vi "Verify Cancel.vi"(11 "Calling VI":refnum<vi>) -> (0 "error out":errorcluster, 2 "Close IE":bool)   [LabVIEW 2020, in "lv_icon.lvlib"]
doc: "Checks if there were changes to the icon and allows the user to select to keep or discord those changes or to return to the Icon Editor."
uses:
  lv_icon.lvlib
  History/History.lvclass
  Controls/Undo Redo Action.ctl
panel:
  in  "Cancel":bool
  in  "Discard":bool
  in  "Apply":bool
  # "The icon has unapplied changes.\nDo you want to apply or discard the changes?"
  # "Apply the changes to the VI"
  # "Changes are discarded and the Icon Editor will be closed"
  # "Return to the Icon Editor"
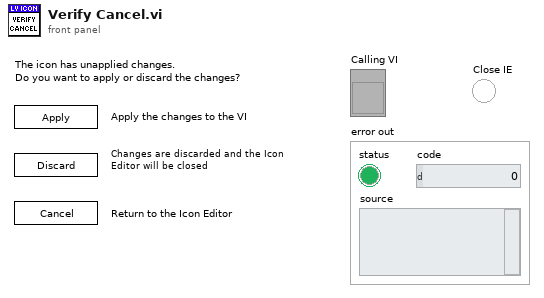
[diagram p1: front panel]
types:
  T1 = typedef "Undo Redo Action.ctl" = enum16{"Init", "Add", "Undo", "Redo", "Current State"}
  T2 = enum32{"Invalid", "Standard", "Closed", "Hidden", "Minimized", "Maximized"}
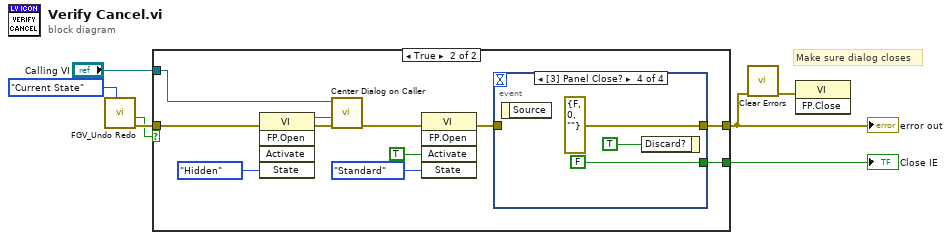
[diagram p0: block diagram]
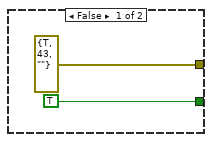
[diagram p2: hidden frame]
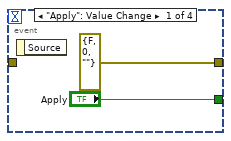
[diagram p3: hidden frame]
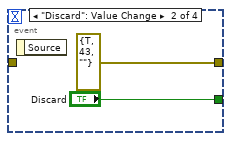
[diagram p4: hidden frame]
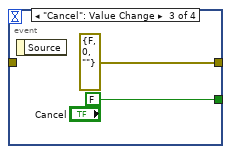
[diagram p5: hidden frame]
diagram:
  # "Make sure dialog closes"
  n1 = call "FGV_Undo Redo.vi"("Action"=Undo_Redo_Action."Current State") -> ("error out"=w7:errorcluster, "Have Changes"=w3:bool)  [unwired: 8 in, 1 out]
  n2 = case shown="True" w3 {
    tunnel: w7 -> [_ w20]
    tunnel: [errorcluster {"status"=TRUE, "code"=43, "source"=""} ("error out") w19] -> w5
    tunnel: [TRUE ("Cancel") w15] -> w2
    tunnel: "Calling VI" -> [_ w11]
    frame False {
    }
    frame True {
      n3 = invoke class="VI" method="FP.Open"(error in=w20, "State"=T2."Hidden") -> (reference out=w10:refnum<vi>, error out=w18:errorcluster)  [unwired: 3 in, 3 out]
      n4 = call "Center Dialog on Caller.vi"("error in"=w18, "Dialog VI"=w10, "Calling VI in"=w11) -> ("error out"=w17:errorcluster)  [unwired: 8 in]
      n5 = invoke class="VI" method="FP.Open"(error in=w17, "Activate"=TRUE ("Activate?"), "State"=T2."Standard") -> (error out=w16:errorcluster)  [unwired: 2 in, 4 out]
      n6 = event shown="[3] Panel Close?" {
        selector: _ -> [_ _ _ _]
        dyn-events: _ -> [_ _ _ _]
        timeout: _ -> [_ _ _ _]
        tunnel: [errorcluster {"status"=FALSE, "code"=0, "source"=""} ("error out") errorcluster {"status"=TRUE, "code"=43, "source"=""} ("error out") errorcluster {"status"=FALSE, "code"=0, "source"=""} ("error out") errorcluster {"status"=FALSE, "code"=0, "source"=""} ("error out")] -> w19
        tunnel: ["Apply" "Discard" FALSE ("Discard") FALSE ("Discard")] -> w15
        tunnel: w16 -> [_ _ _ _]
        event "Apply": Value Change {
          n7 = event-data() -> ()  [unwired: 1 in, 1 out]
        }
        event "Discard": Value Change {
          n8 = event-data() -> ()  [unwired: 1 in, 1 out]
        }
        event "Cancel": Value Change {
          n9 = event-data() -> ()  [unwired: 1 in, 1 out]
        }
        event Panel Close? {
          n10 = event-data() -> ()  [unwired: 1 in, 1 out]
          n11 = event-data("Discard?"=TRUE) -> ()  [unwired: 1 in, 1 out]
        }
      }
    }
  }
  "error out" <- w5
  "Close IE" <- w2
  n12 = call <vilib>:"Clear Errors.vi"("error in (no error)"=w5) -> ("error out"=w6:errorcluster)  [unwired: 5 in, 1 out]
  n13 = invoke class="VI" method="FP.Close"(error in=w6) -> ()  [unwired: 2 in, 3 out]
